vi "Check Loop Error.vi"(6 "Exit on Error?":bool, 7 "Ignore Errors":i32[](array[numeric]), 8 "error in (no error)":errorcluster, 11 "Message Queue in":refnum<queue>) -> (0 "error out":errorcluster, 2 "Error?":bool, 3 "Message Queue out":refnum<queue>)   [LabVIEW 2016]
uses:
  Message Queue/Message.ctl
  Message Queue/Enqueue Message (Single).vi
  Message Queue/Message Queue.lvlib
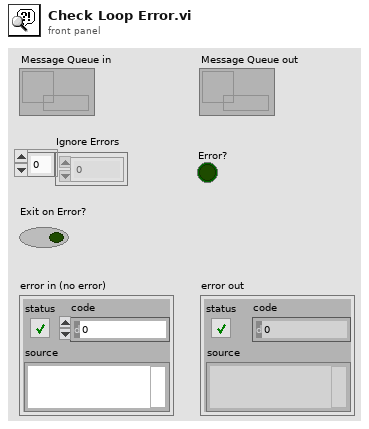
[diagram p1: front panel]
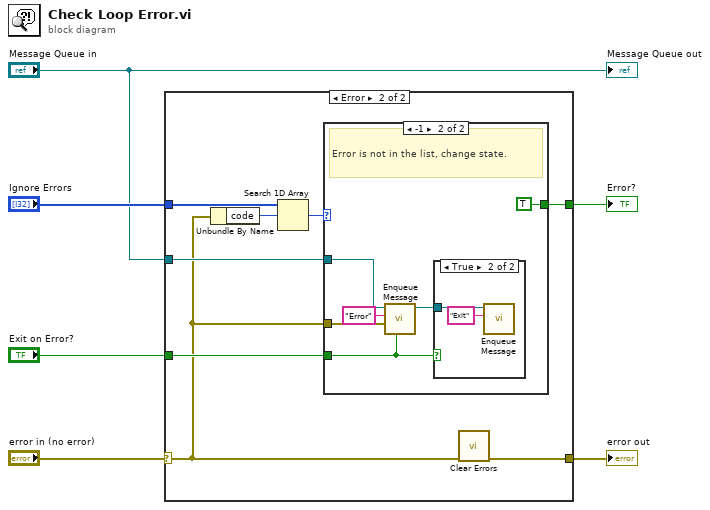
[diagram p0: block diagram]
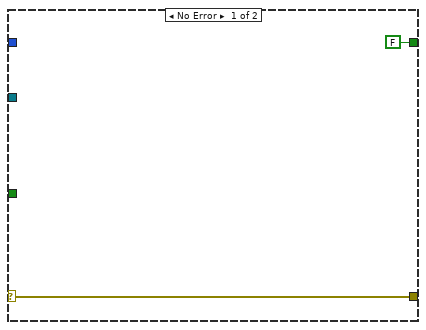
[diagram p2: hidden frame]
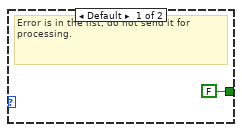
[diagram p3: hidden frame]
diagram:
  n1 = case shown="Error" "error in (no error)" {
    selector: "error in (no error)" -> [w7 w9]
    tunnel: "Ignore Errors" -> [_ w16]
    tunnel: [FALSE w13] -> w4
    tunnel: "Message Queue in" -> [_ w12]
    tunnel: "Exit on Error?" -> [_ w11]
    tunnel: [w7 w10] -> w1
    frame No Error {
    }
    frame Error {
      n2 = Unbundle By Name(w9) -> ("code"=w15:i32)
      n3 = Search 1D Array(1D array=w16, element=w15) -> (index of element=w14:i32)  [unwired: 1 in]
      n4 = case shown="-1" w14 {
        tunnel: w9 -> [_ w21]
        tunnel: [FALSE TRUE] -> w13
        tunnel: w12 -> [_ w22]
        tunnel: w11 -> [_ w19]
        frame Default {
          # "Error is in the list, do not send it for processing."
        }
        frame -1 {
          # "Error is not in the list, change state."
          n5 = call-poly "Enqueue Message.vi"("High Priority?"=w19, "Data"=w21, "State"="Error", "Message Queue in"=w22) -> ("Message Queue out"=w20:refnum<queue>)  [unwired: 6 in, 1 out]
          n6 = case shown="True" w19 {
            tunnel: w20 -> [_ w25]
            frame False {
            }
            frame True {
              n7 = call-poly "Enqueue Message.vi"("State"="Exit", "Message Queue in"=w25) -> ()  [unwired: 8 in, 2 out]
            }
          }
        }
      }
      n8 = call <vilib>:"Clear Errors.vi"("error in (no error)"=w9) -> ("error out"=w10:errorcluster)  [unwired: 5 in, 1 out]
    }
  }
  "Error?" <- w4
  "error out" <- w1
  "Message Queue out" <- "Message Queue in"
